vi "ApplySpectrometerSettings.vi"(8 "error in (no error)":errorcluster, 11 "StellarNetSpecAcquisition in":refnum<class "StellarNetSpecAcquisition.lvclass">) -> (0 "error out":errorcluster, 3 "StellarNetSpecAcquisition out":refnum<class "StellarNetSpecAcquisition.lvclass">)   [LabVIEW 2020, in "StellarNetSpecAcquisition.lvclass"]
uses:
  StellarNetSpecAcquisition.lvclass
  StellarNetSpecAcquisition.lvclass/StellarNetSpecAcquisition.ctl
  StellarNetSpectrometerClass/StellarNetSpectrometer.lvclass
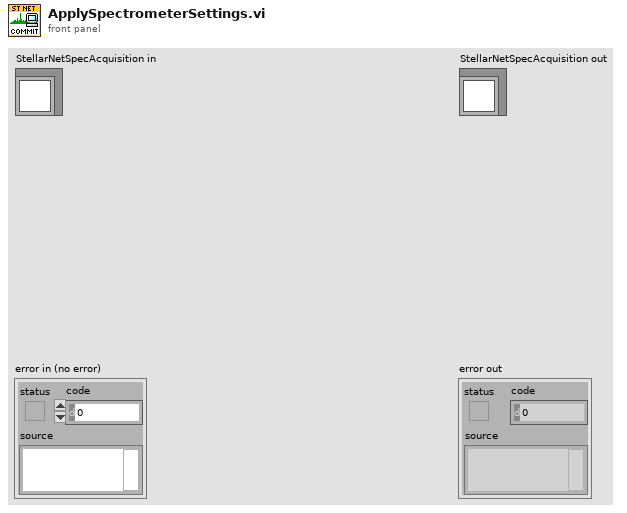
[diagram p1: front panel]
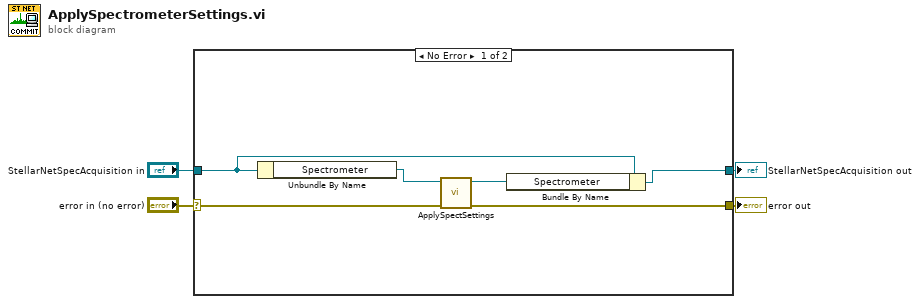
[diagram p0: block diagram]
diagram:
  n1 = case shown="No Error" "error in (no error)" {
    selector: "error in (no error)" -> [w10 w12]
    tunnel: [w9 w12] -> w3
    tunnel: [w7 w11] -> w1
    tunnel: "StellarNetSpecAcquisition in" -> [w8 w11]
    frame No Error {
      n2 = Unbundle By Name(w8) -> ("Spectrometer"=w5:refnum<class "StellarNetSpectrometer.lvclass">)
      n3 = call-dynamic "ApplySpectSettings.vi"("error in"=w10, "StellarNetSpectrometer in"=w5) -> ("error out"=w9:errorcluster, "StellarNetSpectrometer out"=w6:refnum<class "StellarNetSpectrometer.lvclass">)  [unwired: 8 in]
      n4 = Bundle By Name(cluster=w8, "Spectrometer"=w6) -> (w7:refnum<class "StellarNetSpecAcquisition.lvclass">)
    }
    frame Error {
    }
  }
  "error out" <- w3
  "StellarNetSpecAcquisition out" <- w1
